vi "TCP Send Ophir Range.vi"(8 "error in":errorcluster, 11 "Range in":i32) -> (0 "error out":errorcluster, 3 "Range out":i32)   [LabVIEW 2013]
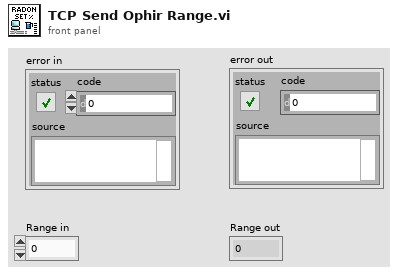
[diagram p1: front panel]
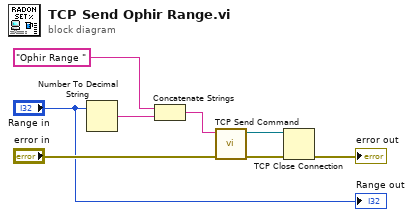
[diagram p0: block diagram]
diagram:
  n1 = Number To Decimal String(number="Range in") -> (decimal integer string=w2:string)  [unwired: 1 in]
  n2 = Concatenate Strings("Ophir Range " ("Command"), w2) -> (w6:string)
  n3 = call "TCP Send Command.vi"("error in"="error in", "Command"=w6) -> ("error out"=w5:errorcluster, "connection ID out"=w3:refnum<k5>)  [unwired: 8 in]
  n4 = TCP Close Connection(connection ID=w3, error in (no error)=w5) -> (error out=→"error out":errorcluster)  [unwired: 1 in, 1 out]
  "Range out" <- "Range in"
